vi "WaveformDBLtoint.vi"(11 "Waveform":waveform(dbl)) -> (0 "32bit integer":i16[](array[numeric]), 1 "scale":dbl, 2 "offset":dbl format="%0.2f", 3 "waveform out":waveform(dbl))   [LabVIEW 2011]
panel:
  out "Waveform 2":waveform(dbl)(graph)
  out "Waveform 2":waveform(dbl)(graph)
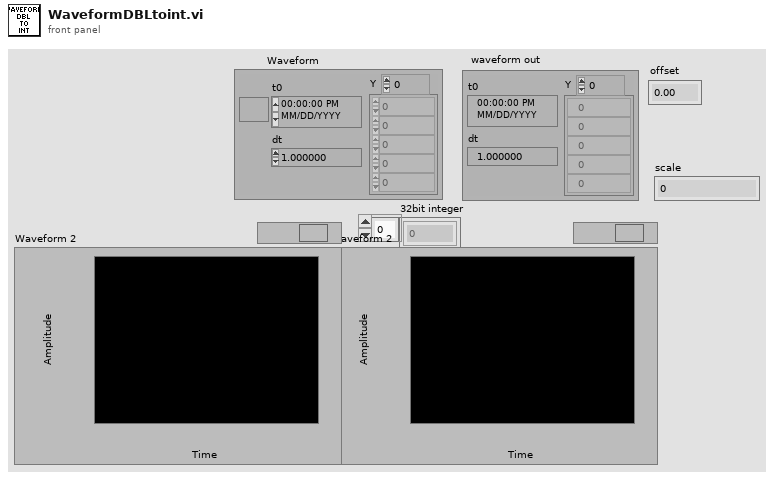
[diagram p1: front panel]
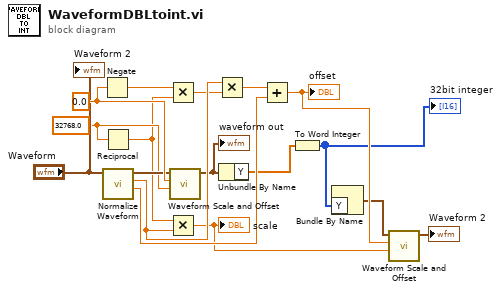
[diagram p0: block diagram]
diagram:
  w13 = 32768.0
  w17 = 0.0 ("offset")
  n1 = Negate(x=w17) -> (-x=w14:dbl)
  n2 = Reciprocal(x=w13) -> (1/x=w12:dbl)
  n3 = call "Normalize Waveform.vi"("waveform in"="Waveform") -> ("offset"=w8:dbl, "scale"=w11:dbl, "normalized waveform"=w16:waveform(dbl))  [unwired: 7 in, 1 out]
  n4 = Multiply(x=w14, y=w12) -> (x*y=w10:dbl)
  n5 = Multiply(x=w12, y=w11) -> (x*y=w6:dbl)
  "scale" <- w6
  n6 = call "Waveform Scale and Offset.vi"("scale"=w13, "offset"=w17, "waveform in"=w16) -> ("waveform out"=w4:waveform(dbl))  [unwired: 7 in, 1 out]
  "waveform out" <- w4
  n7 = Multiply(x=w11, y=w10) -> (x*y=w9:dbl)
  n8 = Unbundle By Name(w4) -> ("Y"=w2:dbl[])
  n9 = Add(x=w9, y=w8) -> (x+y=w7:dbl)
  "offset" <- w7
  n10 = To Word Integer(number=w2) -> (16bit integer=w1:i16[])
  "32bit integer" <- w1
  n11 = Bundle By Name("Y"=w1) -> (w3:waveform(i16))  [unwired: 1 in]
  n12 = call "Waveform Scale and Offset.vi"("scale"=w6, "offset"=w7, "waveform in"=w3) -> ("waveform out"=→"Waveform 2":waveform(dbl))  [unwired: 7 in, 1 out]
  "Waveform 2" <- "Waveform"
